vi "run.hostToFpga.bats.parser.tests.vi"() -> (3 "All Passed?":bool)   [LabVIEW 2022 SP3]
panel:
  out "Results":cluster{"Test Name":string, "Passed?":bool}[](array[cluster])
  out "# of Passed Tests":i32
  out "Seconds":u32
  out "Minutes":u32
  out "# of Test Results":i32
  out "Get All Control\nValues Variant":T1(array[cluster])
  out "error out":errorcluster
  in  "error in":errorcluster
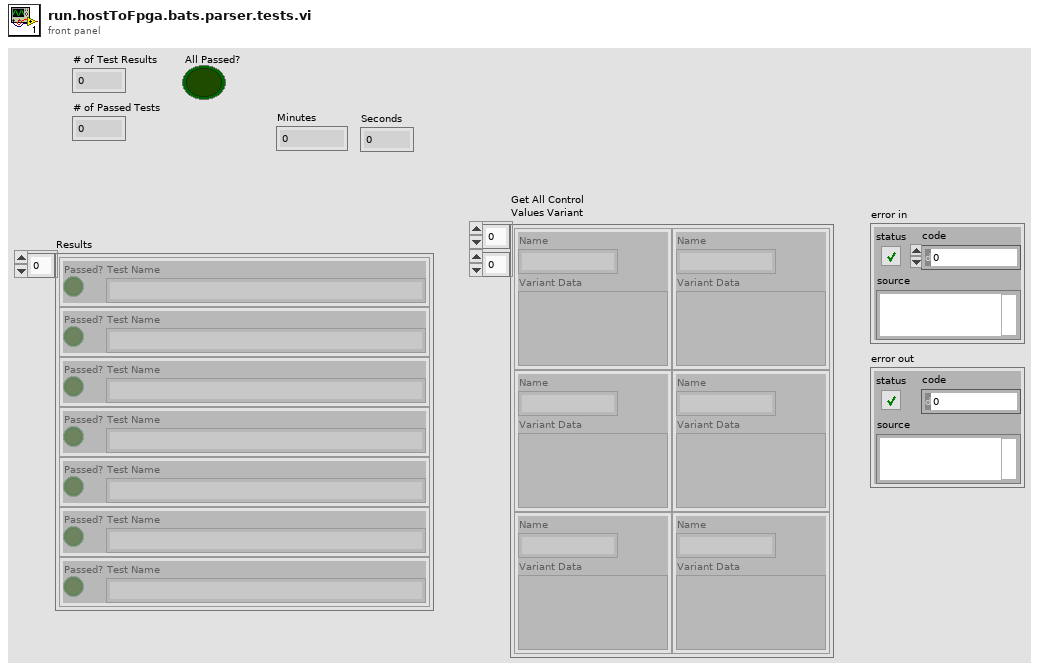
[diagram p1: front panel]
types:
  T1 = cluster{"Name":string, "Variant Data":variant}[][]
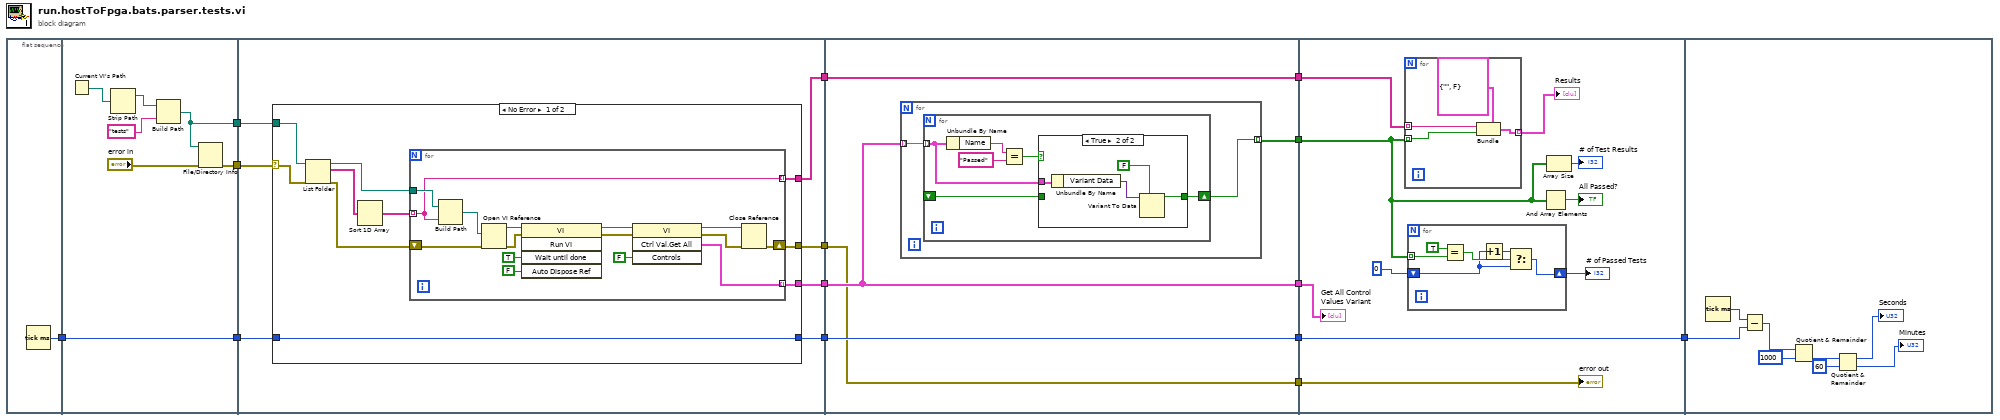
[diagram p0: block diagram]
diagram:
  n1 = flat-sequence {
    tunnel: [w15] -> w11
    tunnel: [w18] -> w14
    tunnel: [w17] -> w13
    tunnel: [w16] -> w12
    tunnel: w11 -> [w16]
    tunnel: w14 -> [w25]
    tunnel: w13 -> [w24]
    tunnel: w12 -> [w23]
    tunnel: [w29] -> w10
    tunnel: [w28] -> w9
    tunnel: [w27] -> w8
    tunnel: [w26] -> w7
    tunnel: w10 -> [w57]
    tunnel: w9 -> [w58]
    tunnel: w8 -> [w61]
    tunnel: w7 -> [w60]
    tunnel: [w61] -> w6
    tunnel: [w60] -> w5
    tunnel: [w59] -> w4
    tunnel: [w58] -> w3
    tunnel: [w57] -> w2
    tunnel: w6 -> [w82]
    tunnel: w5 -> [w84]
    tunnel: w4 -> [w78]
    tunnel: w3 -> [w83]
    tunnel: w2 -> [w79]
    tunnel: [w84] -> w1
    tunnel: w1 -> [w101]
    frame #0 {
      n2 = Tick Count (ms)() -> (millisecond timer value=w15:u32)
    }
    frame #1 {
      n3 = Current VI's Path() -> (path=w21:path)
      n4 = Strip Path(path=w21) -> (stripped path=w22:path)  [unwired: 1 out]
      n5 = Build Path(base path=w22, name or relative path="tests") -> (appended path=w17:path)
      n6 = File/Directory Info(path=w17, error in="error in") -> (error out=w18:errorcluster)  [unwired: 6 out]
    }
    frame #2 {
      n7 = case shown="No Error" w25 {
        selector: w25 -> [w38 w56]
        tunnel: w24 -> [w39 _]
        tunnel: [w36 _] -> w27
        tunnel: [w34 w56] -> w29
        tunnel: [w33 _] -> w28
        tunnel: w23 -> [w32 w55]
        tunnel: [w32 w55] -> w26
        frame No Error {
          n8 = List Folder(path=w39, error in=w38) -> (path out=w37:path, filenames=w31:string[], error out=w35:errorcluster)  [unwired: 2 in, 1 out]
          n9 = Sort 1D Array(array=w31) -> (sorted array=w30:string[])
          n10 = for {
            tunnel: [w40] -> w36 mode=indexing
            tunnel: w37 -> [w54]
            shift-right: [w50] -> w34
            shift-left: w35 -> [w52]
            tunnel: w30 -> [w40] mode=indexing
            tunnel: [w41] -> w33 mode=indexing
            n11 = Build Path(base path=w54, name or relative path=w40) -> (appended path=w53:path)
            n12 = Open VI Reference(vi path=w53, error in (no error)=w52) -> (vi reference=w51:refnum<vi>, error out=w49:errorcluster)  [unwired: 4 in]
            n13 = invoke class="VI" method="Run VI"(reference=w51, error in=w49, "Wait until done"=TRUE ("Wait Until Done"), "Auto Dispose Ref"=FALSE ("Auto Dispose Reference")) -> (reference out=w48:refnum<vi>, error out=w43:errorcluster)  [unwired: 1 in, 3 out]
            n14 = invoke class="VI" method="Ctrl Val.Get All"(reference=w48, error in=w43, "Controls"=FALSE) -> (reference out=w44:refnum<vi>, error out=w42:errorcluster, "Get All Control Values Variant"=w41:cluster{"Name":string, "Variant Data":variant}[])  [unwired: 1 in, 1 out]
            n15 = Close Reference(reference=w44, error in (no error)=w42) -> (error out=w50:errorcluster)
          }
        }
        frame Error {
        }
      }
    }
    frame #3 {
      n16 = for {
        tunnel: w58 -> [w63] mode=indexing
        tunnel: [w62] -> w59 mode=indexing
        n17 = for {
          tunnel: w63 -> [w66] mode=indexing
          shift-right: [w65] -> w62
          shift-left: _ -> [w64]
          n18 = Unbundle By Name(w66) -> ("Name"=w69:string)
          n19 = Equal?(x=w69, y="Passed") -> (x = y?=w67:bool)
          n20 = case shown="True" w67 {
            tunnel: w66 -> [_ w74]
            tunnel: [w70 w71] -> w65
            tunnel: w64 -> [w70 _]
            frame False {
            }
            frame True {
              n21 = Unbundle By Name(w74) -> ("Variant Data"=w73:variant)
              n22 = Variant To Data(type=FALSE, Variant=w73) -> (data=w71:bool)  [unwired: 1 in, 1 out]
            }
          }
        }
      }
    }
    frame #4 {
      n23 = for {
        tunnel: w82 -> [w94] mode=indexing
        tunnel: w78 -> [w93] mode=indexing
        tunnel: [w92] -> w75 mode=indexing
        n24 = Bundle(cluster=cluster{"Test Name":string, "Passed?":bool} {"Test Name"="", "Passed?"=FALSE}, "Test Name"=w94, "Passed?"=w93) -> (w92:cluster{"Test Name":string, "Passed?":bool})
      }
      "Results" <- w75
      n25 = for {
        tunnel: w78 -> [w90] mode=indexing
        shift-right: [w87] -> w76
        shift-left: 0 -> [w86]
        n26 = Equal?(x=TRUE, y=w90) -> (x = y?=w88:bool)
        n27 = Increment(x=w86) -> (x+1=w85:i32)
        n28 = Select(t=w85, s=w88, f=w86) -> (s? t:f=w87:i32)
      }
      "# of Passed Tests" <- w76
      n29 = And Array Elements(Boolean array=w78) -> (logical AND=→"All Passed?":bool)
      n30 = Array Size(array=w78) -> (size(s)=→"# of Test Results":i32)
      "Get All Control\nValues Variant" <- w83
      "error out" <- w79
    }
    frame #5 {
      n31 = Tick Count (ms)() -> (millisecond timer value=w102:u32)
      n32 = Subtract(x=w102, y=w101) -> (x-y=w100:u32)
      n33 = Quotient & Remainder(x=w100, y=u32 1000) -> (floor(x/y)=w98:u32)  [unwired: 1 out]
      n34 = Quotient & Remainder(x=w98, y=u32 60) -> (x-y*floor(x/y)=→"Seconds":u32, floor(x/y)=→"Minutes":u32)
    }
  }
